vi "Read Parent Attributes.vi"(11 "Base Actor in":refnum<class "Base Actor.lvclass">) -> (2 "Parent Attributes":refnum<data-value>)   [LabVIEW 2020, in "jettl.lvlib" / "Base jettl Actor.lvlib" / "Base Actor.lvlib" / "Base Actor.lvclass"]
uses:
  Base Actor.lvclass
  Base Actor.lvclass/Base Actor.ctl
  Transport/Transport.lvclass
  Msg/Msg.lvclass
  Msgs.ctl
  jettl.lvlib
  Actor/Actor.lvclass
  Attributes Metadata/Attributes Metadata.lvclass
  Attributes.ctl
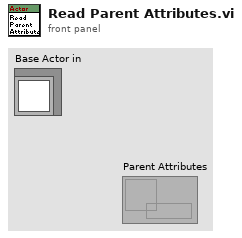
[diagram p1: front panel]
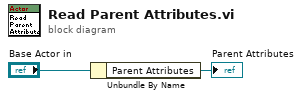
[diagram p0: block diagram]
diagram:
  n1 = Unbundle By Name("Base Actor in") -> ("Parent Attributes"=→"Parent Attributes":refnum<data-value>)
